vi "Untitled 2.vi"() -> ()   [LabVIEW 2015]
uses:
  <vilib>/DAQmx/read.llb/DAQmx Read (Analog DBL 1Chan 1Samp).vi
  <vilib>/DAQmx/create/channels.llb/DAQmx Create Channel (AI-Voltage-Basic).vi
  <vilib>/DAQmx/miscellaneous.llb/DAQmx Fill In Error Info.vi
panel:
  in  "physical channels":tag
  in  "name to assign":string
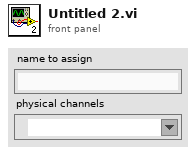
[diagram p1: front panel]
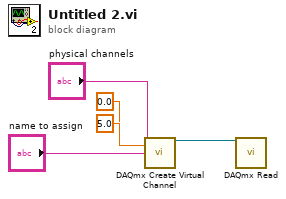
[diagram p0: block diagram]
diagram:
  n1 = call-poly <vilib>:"DAQmx Create Virtual Channel.vi"("maximum value"=5.0, "minimum value"=0.0, "physical channels"="physical channels", "name to assign"="name to assign") -> ("task out"=w5:refnum<k21>)  [unwired: 10 in, 1 out]
  n2 = call-poly <vilib>:"DAQmx Read.vi"("task/channels in"=w5) -> ()  [unwired: 12 in, 3 out]
